vi "MGI Milliseconds Since Last Reset.vi"(6 "Reset (F)":bool, 7 "Error In":errorcluster) -> (2 "ms":u32, 3 "Error Out":errorcluster)   [LabVIEW 2020]
doc: "Returns the amount of time in milliseconds since the last time the VI was reset. This VI is non-reentrant.\n\nAuthored by Brandon D. Steele\nsupport@mooregoodideas.com\nwww.mooregoodideas.com\n\nCopyright (c) 2010, Moore Good Ideas, Inc.\n\nAll rights reserved.\n\nRedistribution and use in source and binary forms, with or without modification, are permitted provided that the following conditions are met:\n\n * Redistributions of source code must retain the above copyright notice, this list of conditions and the following disclaimer.\n * Redistributions in binary form must reproduce the above copyright notice, this list of conditions and the following disclaimer in the documentation and/or other materials provided with the distribution.\n * Neither the name of Moore Good Ideas, Inc. nor the names of its contributors may be used to endorse or promote products derived from this software without specific prior written permission.\n\nTHIS SOFTWARE IS PROVIDED BY THE COPYRIGHT HOLDERS AND CONTRIBUTORS \"AS IS\" AND ANY EXPRESS OR IMPLIED WARRANTIES, INCLUDING, BUT NOT LIMITED TO, THE IMPLIED WARRANTIES OF MERCHANTABILITY AND FITNESS FOR A PARTICULAR PURPOSE ARE DISCLAIMED. IN NO EVENT SHALL THE COPYRIGHT OWNER OR CONTRIBUTORS BE LIABLE FOR ANY DIRECT, INDIRECT, INCIDENTAL, SPECIAL, EXEMPLARY, OR CONSEQUENTIAL DAMAGES (INCLUDING, BUT NOT LIMITED TO, PROCUREMENT OF SUBSTITUTE GOODS OR SERVICES; LOSS OF USE, DATA, OR PROFITS; OR BUSINESS INTERRUPTION) HOWEVER CAUSED AND ON ANY THEORY OF LIABILITY, WHETHER IN CONTRACT, STRICT LIABILITY, OR TORT (INCLUDING NEGLIGENCE OR OTHERWISE) ARISING IN ANY WAY OUT OF THE USE OF THIS SOFTWARE, EVEN IF ADVISED OF THE POSSIBILITY OF SUCH DAMAGE."
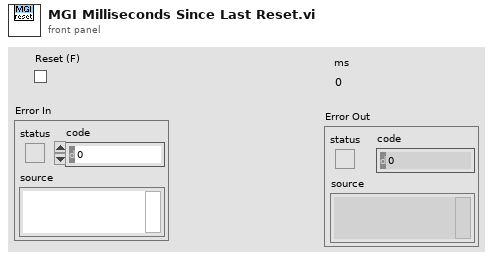
[diagram p1: front panel]
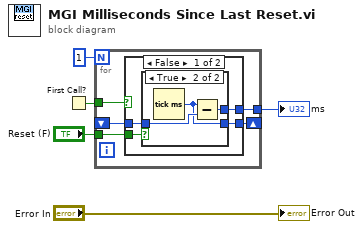
[diagram p0: block diagram]
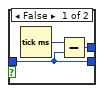
[diagram p2: hidden frame]
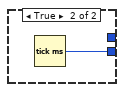
[diagram p3: hidden frame]
diagram:
  n1 = First Call?() -> (First Call?: T/F=w3:bool)
  n2 = for {
    N: 1 -> [_]
    shift-right: [w10] -> _
    shift-left: _ -> [w9]
    tunnel: [w8] -> w4
    tunnel: "Reset (F)" -> [w7]
    tunnel: w3 -> [w6]
    n3 = case shown="False" w6 {
      tunnel: [w14 w21] -> w10
      tunnel: w9 -> [w13 _]
      tunnel: [w12 _] -> w8
      tunnel: w7 -> [w11 _]
      frame False {
        n4 = case shown="True" w11 {
          tunnel: [w15 w18] -> w14
          tunnel: w13 -> [w15 w19]
          tunnel: [w17 w20] -> w12
          frame False {
            n5 = Tick Count (ms)() -> (millisecond timer value=w16:u32)
            n6 = Subtract(x=w16, y=w15) -> (x-y=w17:u32)
          }
          frame True {
            n7 = Tick Count (ms)() -> (millisecond timer value=w18:u32)
            n8 = Subtract(x=w18, y=w19) -> (x-y=w20:u32)
          }
        }
      }
      frame True {
        n9 = Tick Count (ms)() -> (millisecond timer value=w21:u32)
      }
    }
  }
  "ms" <- w4
  "Error Out" <- "Error In"
